vi "Remove Bracketed characters.vi"(0 "Input String":string, 1 "Max String Length (0)":i32) -> (2 "audit":string[](array[string]), 3 "Output String":string, 4 "finalLength":i32, 5 "stillTooLong":bool)   [LabVIEW 2022 SP3]
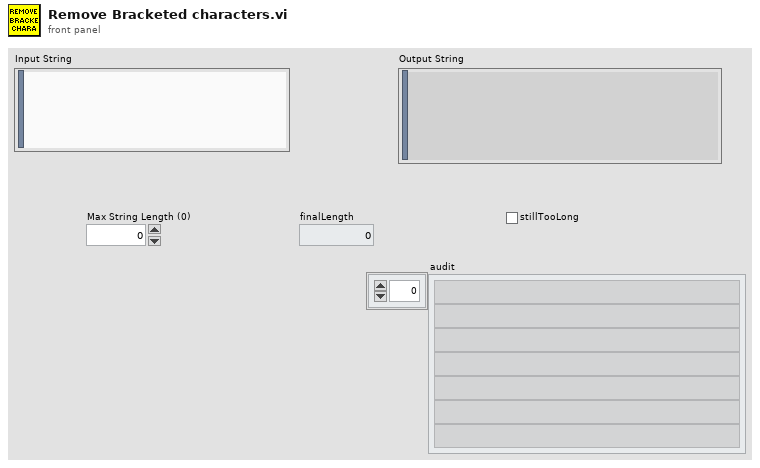
[diagram p1: front panel]
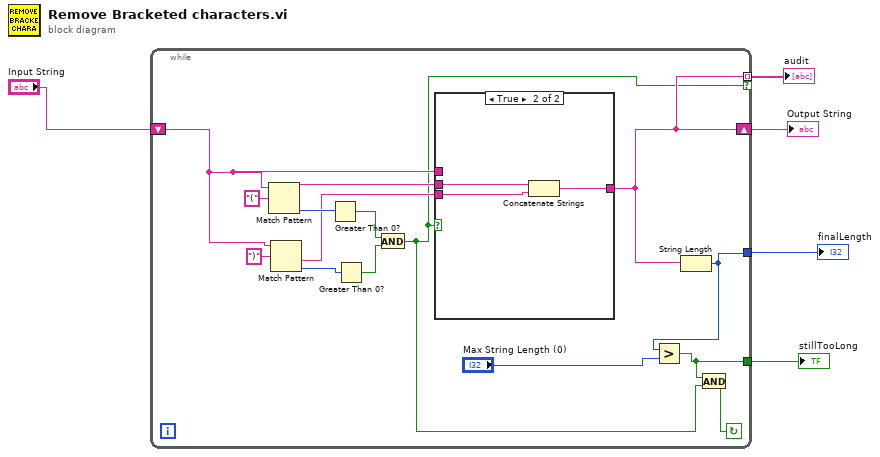
[diagram p0: block diagram]
diagram:
  n1 = while {
    shift-right: [w11] -> w5
    shift-left: "Input String" -> [w12]
    tunnel: [w11] -> w3 mode=indexing if=w8
    tunnel: [w10] -> w2
    tunnel: [w6] -> w1
    stop <- w7 continue-if-true
    n2 = Match Pattern(string=w12, regular expression="(") -> (before substring=w14:string, offset past match=w18:i32)  [unwired: 1 in, 2 out]
    n3 = Match Pattern(string=w12, regular expression=")") -> (after substring=w13:string, offset past match=w17:i32)  [unwired: 1 in, 2 out]
    n4 = Greater Than 0?(x=w18) -> (x > 0?=w15:bool)
    n5 = Greater Than 0?(x=w17) -> (x > 0?=w16:bool)
    n6 = And(x=w15, y=w16) -> (x .and. y?=w8:bool)
    n7 = case shown="True" w8 {
      tunnel: w14 -> [_ w24]
      tunnel: w13 -> [_ w23]
      tunnel: [w21 w22] -> w11
      tunnel: w12 -> [w21 _]
      frame False {
      }
      frame True {
        n8 = Concatenate Strings(w24, w23) -> (w22:string)
      }
    }
    n9 = String Length(string=w11) -> (length=w10:i32)
    n10 = Greater?(x=w10, y="Max String Length (0)") -> (0:w6:bool)
    n11 = And(x=w6, y=w8) -> (x .and. y?=w7:bool)
  }
  "Output String" <- w5
  "audit" <- w3
  "stillTooLong" <- w1
  "finalLength" <- w2
